vi "GreaterThan.vi"(0 "A":T1={"Array Num"=[1, 2, 3], "Decimal Index"=0, "stop"=FALSE}, 1 "B":T1={"Array Num"=[1, 2, 3], "Decimal Index"=0, "stop"=FALSE}) -> (2 "Larger":T1={"Array Num"=[1, 2, 3], "Decimal Index"=0, "stop"=FALSE}, 3 "Smaller":T1={"Array Num"=[1, 2, 3], "Decimal Index"=0, "stop"=FALSE}, 4 "A Greater":bool, 5 "Equal":bool)   [LabVIEW 2025]
doc: "Doesn't work with sign of numbers yet."
uses:
  Number.ctl
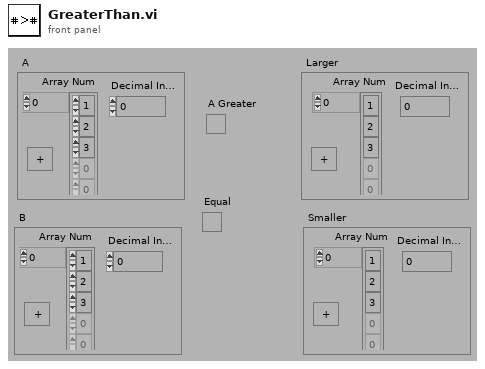
[diagram p1: front panel]
types:
  T1 = typedef "Number.ctl" = cluster{"Array Num":i8[], "Decimal Index":i32, "stop":bool}
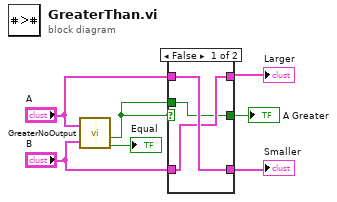
[diagram p0: block diagram]
diagram:
  n1 = call "GreaterNoOutput.vi"("A"="A", "B"="B") -> ("A Greater"=w2:bool, "Equal"=→"Equal":bool)  [unwired: 1 in, 1 out]
  n2 = case shown="False" w2 {
    tunnel: "A" -> [w10 w13]
    tunnel: "B" -> [w9 w12]
    tunnel: [w10 w12] -> w5
    tunnel: [w9 w13] -> w6
    tunnel: [w8 w11] -> w7
    tunnel: w2 -> [w8 w11]
    frame False {
    }
    frame True {
    }
  }
  "A Greater" <- w7
  "Larger" <- w6
  "Smaller" <- w5
